vi "Local Dir to FTP Dir.vi"(7 "Root Path":path, 8 "error in (no error)":errorcluster, 10 "Path":path, 11 "FTPProtocol in":refnum<class "FTPProtocol.lvclass">) -> (0 "error out":errorcluster, 1 "parent folder in ftp":string, 2 "ftp path":string, 3 "FTPProtocol out":refnum<class "FTPProtocol.lvclass">)   [LabVIEW 2020, in "FileSync -- FTP.lvlib" / "FTPProtocol.lvclass"]
uses:
  FTPProtocol.lvclass
  FTPProtocol.lvclass/FTPProtocol.ctl
  <userlib>/_NEVSTOP/Communicable State Machine(CSM)/_Shared/CSM Shared.lvlib
  <userlib>/_NEVSTOP/Communicable State Machine(CSM)/Communicable State Machine.lvlib
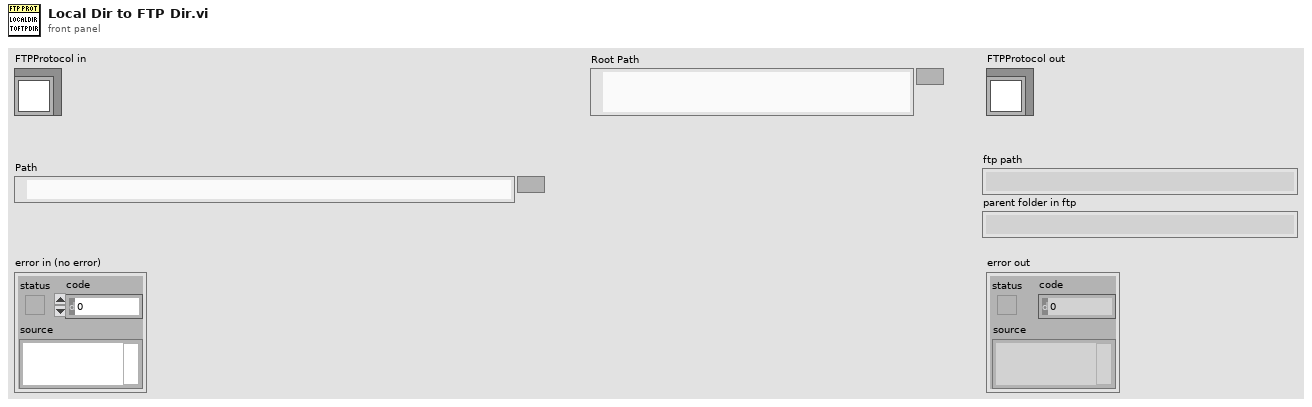
[diagram p1: front panel]
types:
  T1 = cluster{"address":string, "remote port":u16, "userName":string, "passWord":string, "RootDir":string}
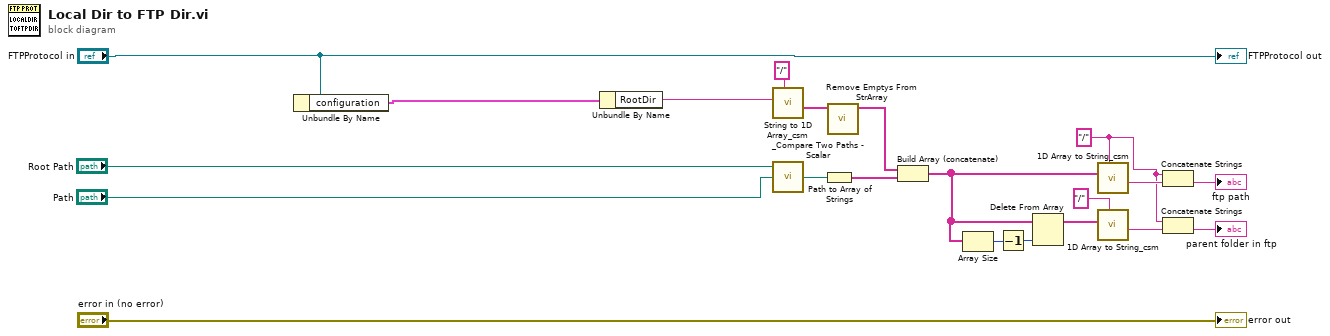
[diagram p0: block diagram]
diagram:
  w5 = "/" ("delimiter (Tab)")
  n1 = Unbundle By Name("FTPProtocol in") -> ("configuration"=w2:T1)
  n2 = Unbundle By Name(w2) -> ("RootDir"=w1:string)
  n3 = call <userlib>:"String to 1D Array_csm.vi"("delimiter (Tab)"="/", "string"=w1) -> ("Array of Strings"=w16:string[])  [unwired: 9 in]
  n4 = call "_Compare Two Paths - Scalar.vi"("path2"="Path", "path1"="Root Path") -> ("relative path from 1 to 2"=w20:path)  [unwired: 1 in, 2 out]
  n5 = Path to Array of Strings(0:w20) -> (2:w4:string[])  [unwired: 1 out]
  n6 = call <userlib>:"Remove Emptys From StrArray.vi"("Array in"=w16) -> ("Array out"=w15:string[])  [unwired: 10 in]
  n7 = Build Array (concatenate)(w15, w4) -> (w11:string[])
  n8 = Array Size(array=w11) -> (size(s)=w12:i32)
  n9 = Decrement(x=w12) -> (x-1=w13:i32)
  n10 = Delete From Array(array=w11, index=w13) -> (array with subset deleted=w9:string[])  [unwired: 1 in, 1 out]
  n11 = call <userlib>:"1D Array to String_csm.vi"("delimiter (Tab)"=w5, "Array of Strings"=w11) -> ("delimited string"=w14:string)  [unwired: 9 in]
  n12 = call <userlib>:"1D Array to String_csm.vi"("delimiter (Tab)"="/", "Array of Strings"=w9) -> ("delimited string"=w8:string)  [unwired: 9 in]
  n13 = Concatenate Strings(w5, w14) -> (→"ftp path":string)
  n14 = Concatenate Strings(w5, w8) -> (→"parent folder in ftp":string)
  "error out" <- "error in (no error)"
  "FTPProtocol out" <- "FTPProtocol in"
